vi "standardize CSM Module.vi"(8 "Error In":errorcluster, 11 "CSM-Helper In":refnum<class "CSM-Helper.lvclass">) -> (0 "error out":errorcluster, 3 "CSM-Helper Out":refnum<class "CSM-Helper.lvclass">)   [LabVIEW 2017, in "CSM-Helper.lvclass"]
doc: "### standardize CSM Module.vi\n\n-- <b>Controls</b> --\n- <b>CSM-Helper in</b>: CSMHelper input\n\n-- <b>Indicators</b> --\n- <b>CSM-Helper out</b>: CSMHelper output"
uses:
  CSM-Helper.lvclass
  CSM-Helper.lvclass/CSM-Helper.ctl
  Properties/Read Type.vi
  API/Set Visible Case Frame.vi
  API/Get CaseFrame Reference By CaseName.vi
  API/Stop Undo.vi
  API/Start Undo.vi
  Utility/CSM-Helper Utility.lvlib
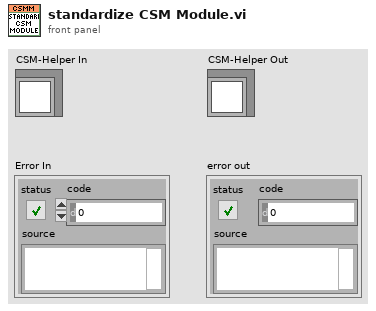
[diagram p1: front panel]
types:
  T1 = enum32{"Invalid", "Standard", "Closed", "Hidden", "Minimized", "Maximized"}
  T2 = enum32{"invalid app kind", "Development System", "Run Time System", "Student Edition", "Embedded LabVIEW", "Evaluation", "Custom"}
  T3 = cluster{"Core":cluster{"Current VI Reference":refnum<vi>, "Close Panel on Exit?":bool}, "Your Boolean data":bool, "Your string data":string}
  T4 = cluster{"Current VI Reference":refnum<vi>, "Close Panel on Exit?":bool}
  T5 = typedef "CSM-Helper Utility.lvlib/CSM Module Type.ctl" = enum16{"Not a CSM", "JKISM", "CSM"}
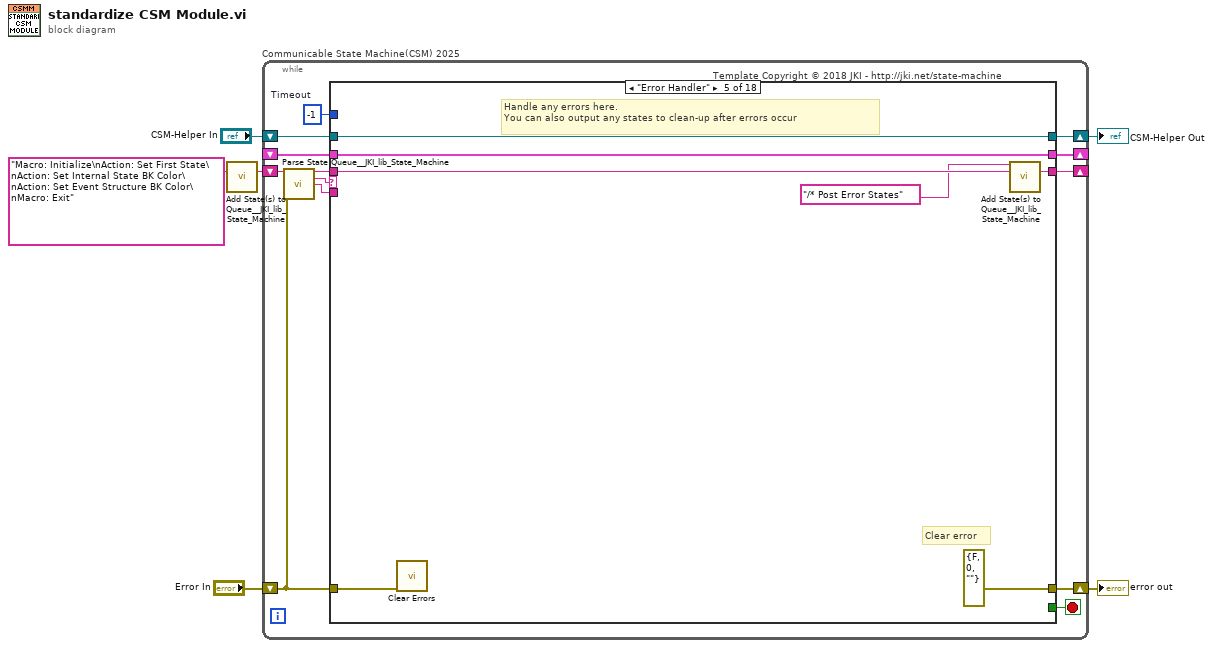
[diagram p0: block diagram]
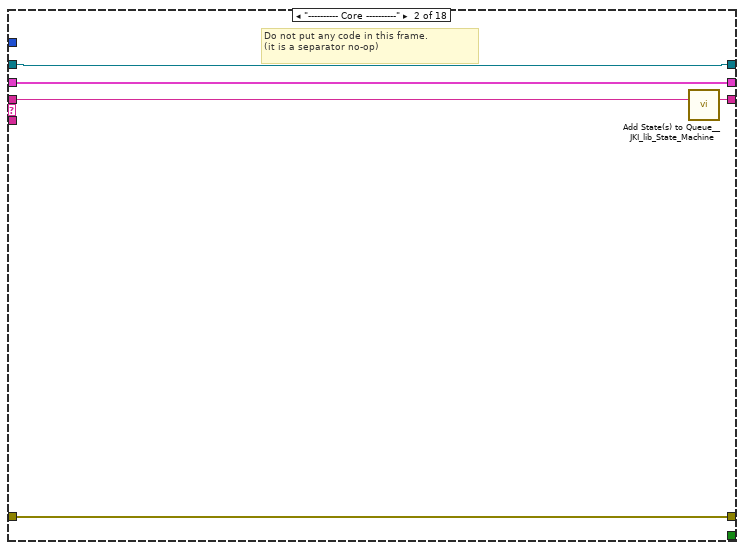
[diagram p3: hidden frame]
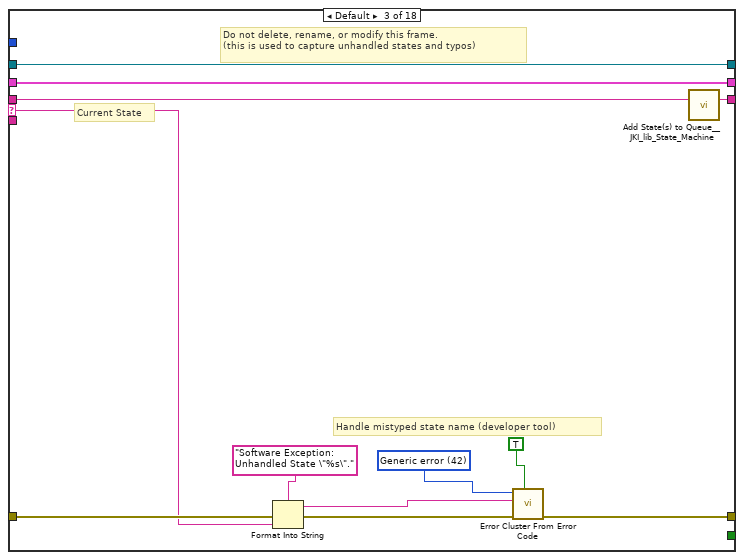
[diagram p4: hidden frame]
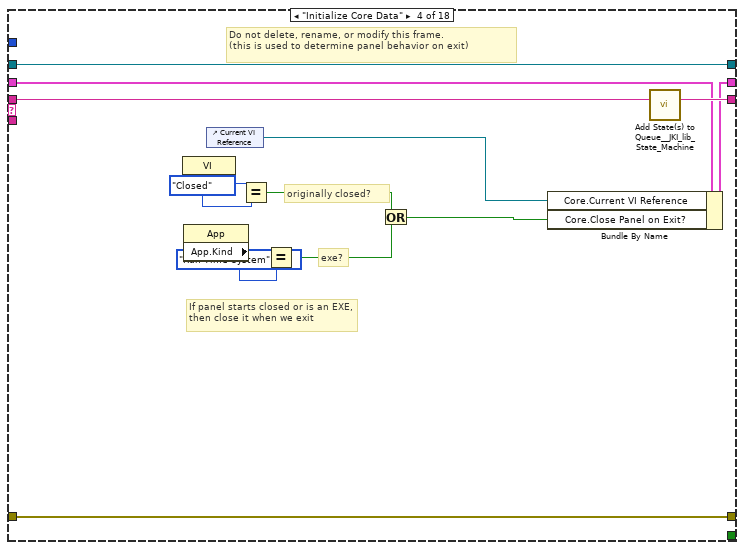
[diagram p5: hidden frame]
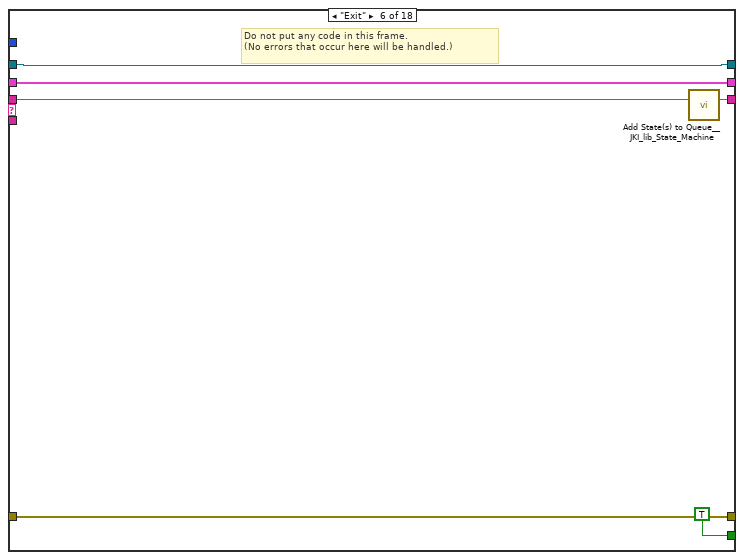
[diagram p6: hidden frame]
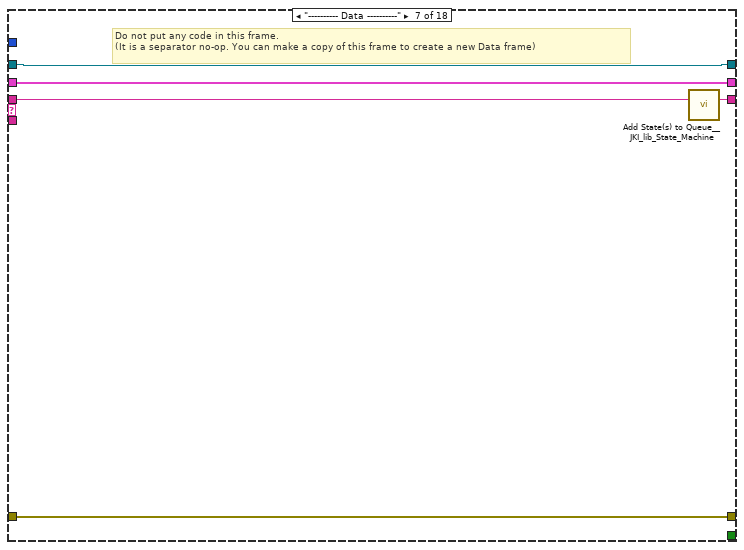
[diagram p7: hidden frame]
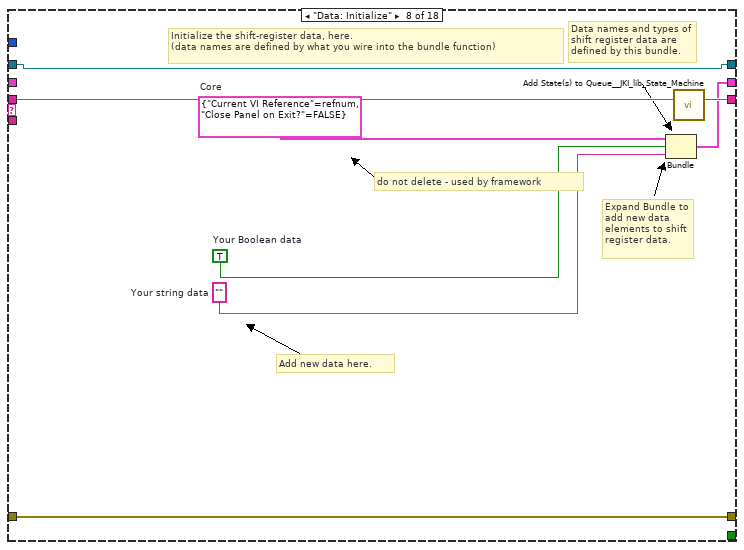
[diagram p8: hidden frame]
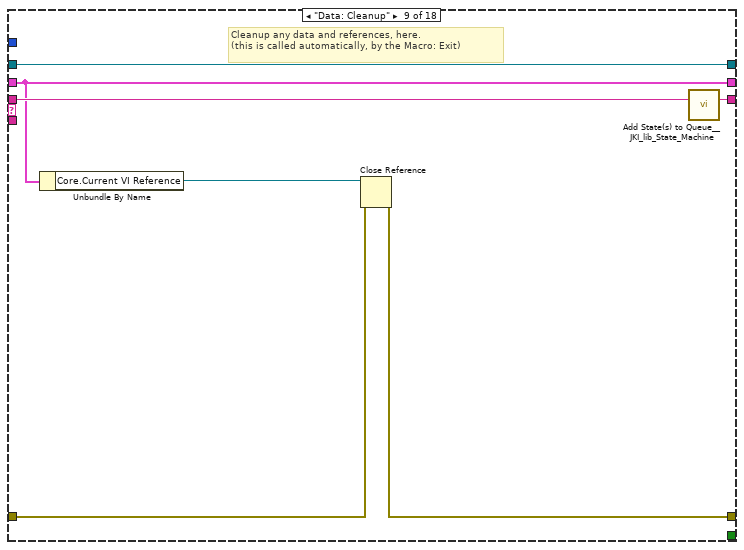
[diagram p9: hidden frame]
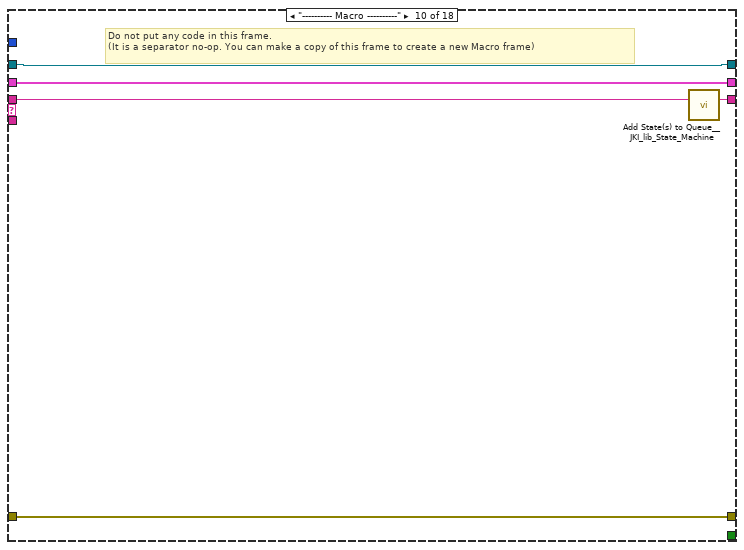
[diagram p10: hidden frame]
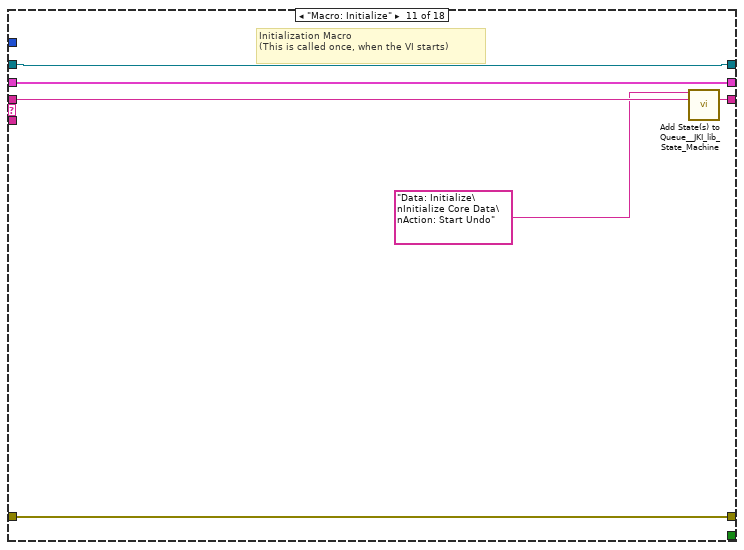
[diagram p11: hidden frame]
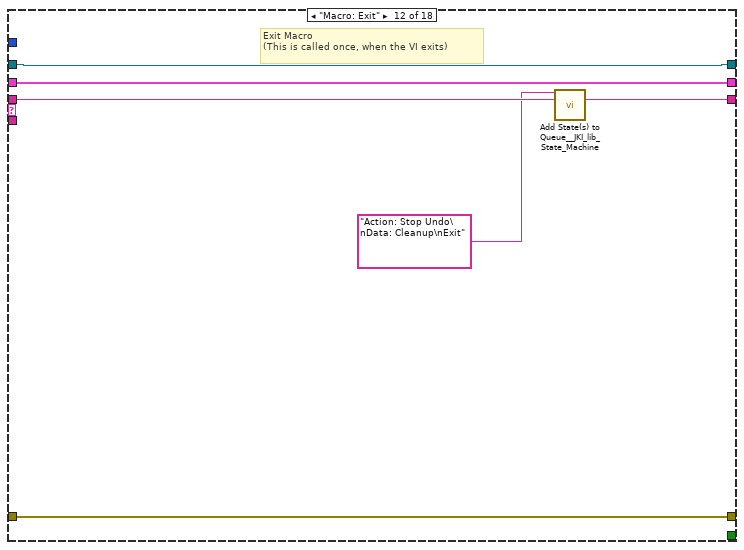
[diagram p12: hidden frame]
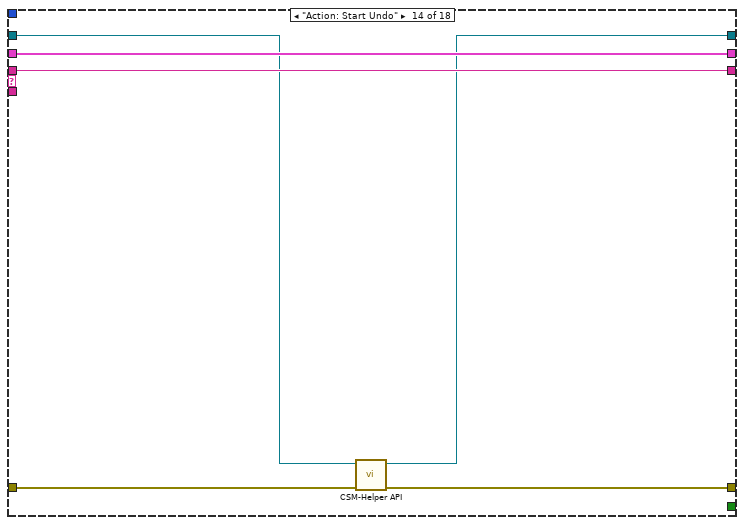
[diagram p14: hidden frame]
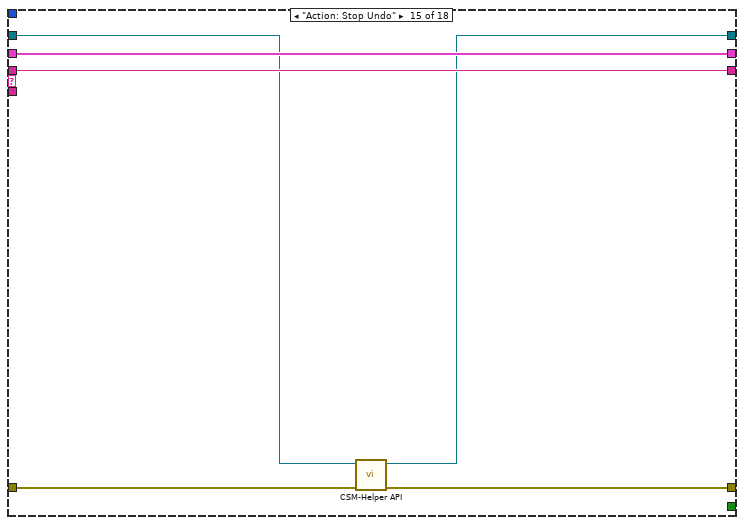
[diagram p15: hidden frame]
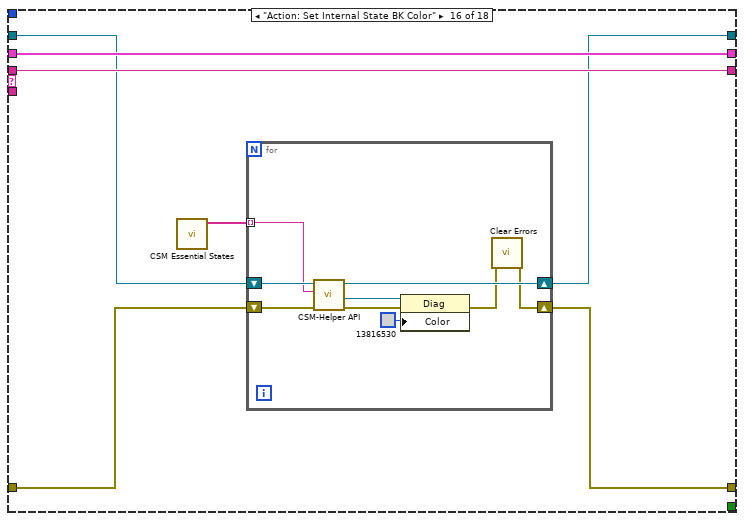
[diagram p16: hidden frame]
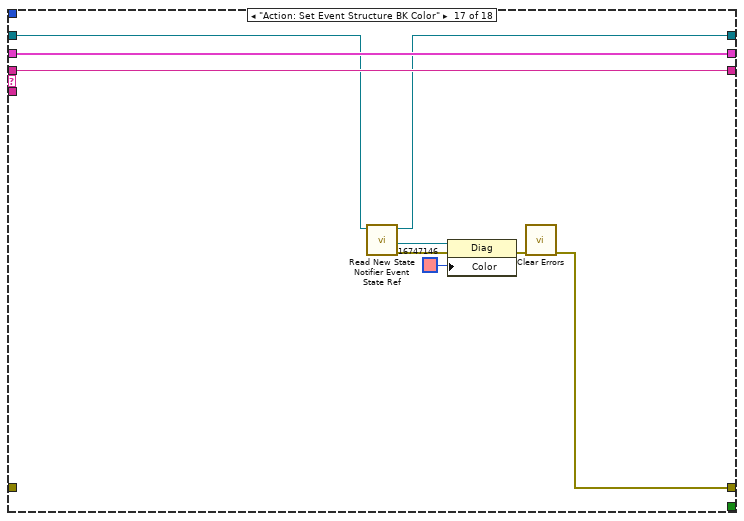
[diagram p17: hidden frame]
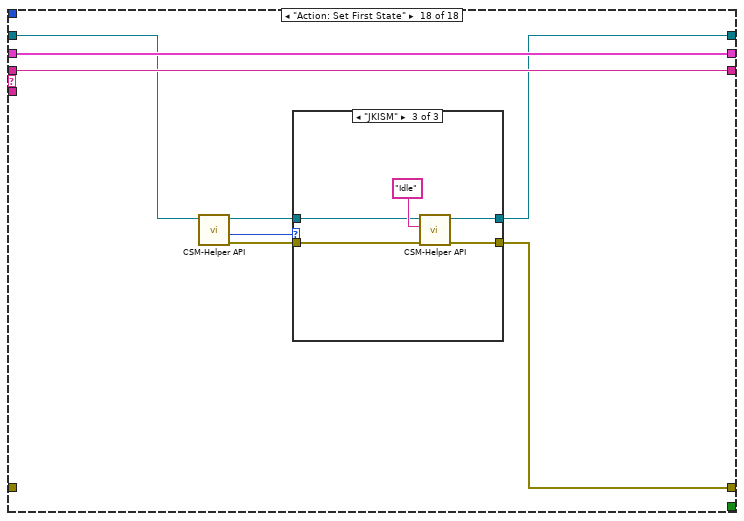
[diagram p18: hidden frame]
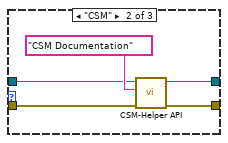
[diagram p20: hidden frame]
diagram:
  n1 = call <vilib>:"Add State(s) to Queue__JKI_lib_State_Machine.vi"("State(s) in (\"\")"="Macro: Initialize\nAction: Set First State\nAction: Set Internal State BK Color\nAction: Set Event Structure BK Color\nMacro: Exit") -> ("States Out"=w6:string)  [unwired: 14 in]
  n2 = while "Communicable State Machine(CSM) 2025" {
    shift-right: [w12] -> _
    shift-left: _ -> [w11]
    shift-right: [w15] -> w3
    shift-left: "Error In" -> [w9]
    shift-right: [w14] -> _
    shift-left: w6 -> [w16]
    shift-right: [w7] -> w1
    shift-left: "CSM-Helper In" -> [w8]
    stop <- w13 stop-if-true
    w10 = -1  # Timeout
    # "Template Copyright © 2018 JKI - http://jki.net/state-machine"
    n3 = call <vilib>:"Parse State Queue__JKI_lib_State_Machine.vi"("State Queue"=w16, "Error In (no error)"=w9) -> ("Remaining States"=w18:string, "Current State"=w19:string, "Arguments"=w17:string)  [unwired: 11 in]
    n4 = case shown="\"Error Handler\"" w19 {
      selector: w19 -> [_ _ w30 _ _ _ _ _ _ _ _ _ _ _ _ _ _ _]
      tunnel: w18 -> [w23 w28 w34 w54 w61 w67 w72 w80 w87 w92 w98 w104 w106 w113 w119 w127 w145 w153]
      tunnel: w17 -> [_ _ _ _ _ _ _ _ _ _ _ _ _ _ _ _ _ _]
      tunnel: w11 -> [w21 w25 w32 w47 w58 w65 w69 _ w82 w89 w95 w101 w107 w114 w120 w126 w144 w152]
      tunnel: [w22 w26 w36 w51 errorcluster {"status"=FALSE, "code"=0, "source"=""} ("error out") w64 w70 w77 w83 w90 w96 w102 w105 w111 w117 w122 w137 w150] -> w15
      tunnel: w9 -> [w22 w26 w35 w51 w57 w64 w70 w77 w84 w90 w96 w102 w105 w112 w118 w123 _ _]
      tunnel: [w23 w27 w33 w53 w60 w66 w71 w79 w86 w91 w97 w103 w106 w113 w119 w127 w145 w153] -> w14
      tunnel: [_ _ _ _ _ TRUE _ _ _ _ _ _ _ _ _ _ _ _] -> w13
      tunnel: [w21 w25 w32 w52 w58 w65 w69 w78 w82 w89 w95 w101 w107 w114 w120 w126 w144 w152] -> w12
      tunnel: w10 -> [_ _ _ _ _ _ _ _ _ _ _ _ _ _ _ _ _ _]
      tunnel: w8 -> [w20 w24 w29 w41 w55 w62 w68 w73 w81 w88 w93 w99 w108 w110 w116 w125 w143 w149]
      tunnel: [w20 w24 w29 w41 w55 w62 w68 w73 w81 w88 w93 w99 w108 w109 w115 w124 w142 w151] -> w7
      frame "", "Event Structure", "Idle" {
        # "executes when the state queue is empty"
      }
      frame "---------- Core ----------" {
        # "Do not put any code in this frame.\n(it is a separator no-op)"
        n5 = call <vilib>:"Add State(s) to Queue__JKI_lib_State_Machine.vi"("State(s) in (\"\")"=w28) -> ("States Out"=w27:string)  [unwired: 14 in]
      }
      frame Default {
        w39 = 42 items=["No error", "Argument error", "Memory is full", "Out of zone", "End of file", "File already open", "Generic file I/O error", "File not found", "File permission error", "Disk is full", "Duplicate path", "Too many files open", "System feature not enabled", "Resource file not found", "Cannot add resource", "Resource not found", "Image not found", "Image memory error", "Pen does not exist", "Config type invalid", "Config token not found", "Config parse error", "Config memory error", "Bad external code format", "Bad external code offset", "External code not present", "Null window", "Destroy window error", "Null menu", "Print aborted", "Bad print record", "Print driver error", "Windows error during printing", "Memory error during printing", "Print dialog error", "Generic print error", "Invalid device refnum", "Device not found", "Device parameter error", "Device unit error", "Cannot open device", "Device call aborted", "Generic error", "Cancelled by user", "Object ID too low", "Object ID too high", "Object not in heap", "Unknown heap", "Unknown object (invalid DefProc)", "Unknown object (DefProc not in table)", "Message out of range", "Invalid (null) method", "Unknown message", "Manager call not supported", "Bad address", "Network operation in progress", "Network operation timed out", "Connection is busy", "Network attribute not supported", "Network error", "Address in use", "System out of memory", "Connection aborted", "Connection refused", "Not connected", "Already connected", "Connection closed", "Initialization error (interapplication manager)", "Bad occurrence", "Wait on unbound occurrence handler", "Occurrence queue overflow", "Datalog type conflict", "Unused", "Unrecognized type (interapplication manager)", "Memory corrupt", "Failed to make temporary DLL", "Old CIN version", "Drag socket not found", "Failed to load drop-object", "Failed to register OLE object", "Failed to release OLE object", "Format specifier type mismatch", "Unknown format specifier", "Too few format specifiers", "Too many format specifiers", "Scan failed", "Newer CIN version", "Error converting to variant", "Runtime menu error", "Password tampered", "Variant attribute not found", "Incompatible variant data type", "Event data is not available", "Event Store is not present", "Occurrence is not found", "Event Queue is not created", "Event info is not available", "Refnum passed is NULL", "Error retrieving Class GUID", "Error retrieving CoClass GUID", "Error retrieving TypeLib GUID.", "Bad built application magic bytes.", "Specific driver is different from the specific driver associated with the Logical Name.", "There is no session opened to the class driver.", "Max Error", "MAX - Error with config objects", "MAX - Error loading configuration", "MAX - Group not supported"]
        # "Current State"
        # "Do not delete, rename, or modify this frame.\n(this is used to capture unhandled states and typos)"
        # "Handle mistyped state name (developer tool)"
        n6 = Format Into String(format string="Software Exception: Unhandled State \"%s\"." ("message"), error in=w35, w30) -> (resulting string=w38:string, error out=w37:errorcluster)  [unwired: 1 in]
        n7 = call <vilib>:"Error Cluster From Error Code.vi"("show call chain? (False)"=TRUE, "error in (no error)"=w37, "error message (\"\")"=w38, "error code (0)"=w39) -> ("error out"=w36:errorcluster)  [unwired: 5 in]
        n8 = call <vilib>:"Add State(s) to Queue__JKI_lib_State_Machine.vi"("State(s) in (\"\")"=w34) -> ("States Out"=w33:string)  [unwired: 14 in]
      }
      frame "Initialize Core Data" {
        # "Do not delete, rename, or modify this frame.\n(this is used to determine panel behavior on exit)"
        # "originally closed?"
        # "exe?"
        # "If panel starts closed or is an EXE, then close it when we exit"
        n9 = property class="VI"() -> ("FP.State"=w44:T1)  [unwired: 2 in, 2 out]
        n10 = property class="App"() -> ("App.Kind"=w50:T2)  [unwired: 2 in, 2 out]
        n11 = control-ref of="Current VI Reference"() -> (w45:refnum<vi>)
        n12 = Equal?(x=w44, y=T1."Closed" ("Front Panel Window:State")) -> (x = y?=w42:bool)
        n13 = Equal?(x=w50, y=T2."Run Time System" ("Application:Kind")) -> (x = y?=w48:bool)
        n14 = Or(x=w42, y=w48) -> (x .or. y?=w46:bool)
        n15 = Bundle By Name(cluster=w47, "Core.Current VI Reference"=w45, "Core.Close Panel on Exit?"=w46) -> (w52:T3)
        n16 = call <vilib>:"Add State(s) to Queue__JKI_lib_State_Machine.vi"("State(s) in (\"\")"=w54) -> ("States Out"=w53:string)  [unwired: 14 in]
      }
      frame "Error Handler" {
        # "Handle any errors here.\nYou can also output any states to clean-up after errors occur"
        # "Clear error"
        n17 = call <vilib>:"Clear Errors.vi"("error in (no error)"=w57) -> ()  [unwired: 5 in, 2 out]
        n18 = call <vilib>:"Add State(s) to Queue__JKI_lib_State_Machine.vi"("State(s) in Front (\"\")"="/* Post Error States", "State(s) in (\"\")"=w61) -> ("States Out"=w60:string)  [unwired: 13 in]
      }
      frame "Exit" {
        # "Do not put any code in this frame.\n(No errors that occur here will be handled.)"
        n19 = call <vilib>:"Add State(s) to Queue__JKI_lib_State_Machine.vi"("State(s) in (\"\")"=w67) -> ("States Out"=w66:string)  [unwired: 14 in]
      }
      frame "---------- Data ----------" {
        # "Do not put any code in this frame.\n(It is a separator no-op. You can make a copy of this frame to create a new Data frame)"
        n20 = call <vilib>:"Add State(s) to Queue__JKI_lib_State_Machine.vi"("State(s) in (\"\")"=w72) -> ("States Out"=w71:string)  [unwired: 14 in]
      }
      frame "Data: Initialize" {
        w74 = T4 {"Current VI Reference"=refnum, "Close Panel on Exit?"=FALSE}  # Core
        w76 = TRUE  # Your Boolean data
        w75 = ""  # Your string data
        # "do not delete - used by framework"
        # "Expand Bundle to add new data elements to shift register data."
        # "Add new data here."
        # "Data names and types of shift register data are defined by this bundle."
        # "Initialize the shift-register data, here.\n(data names are defined by what you wire into the bundle function)"
        n21 = Bundle("Core"=w74, "Your Boolean data"=w76, "Your string data"=w75) -> (w78:T3)  [unwired: 1 in]
        n22 = call <vilib>:"Add State(s) to Queue__JKI_lib_State_Machine.vi"("State(s) in (\"\")"=w80) -> ("States Out"=w79:string)  [unwired: 14 in]
      }
      frame "Data: Cleanup" {
        # "Cleanup any data and references, here.\n(this is called automatically, by the Macro: Exit)"
        n23 = Unbundle By Name(w82) -> ("Core.Current VI Reference"=w85:refnum<vi>)
        n24 = Close Reference(reference=w85, error in (no error)=w84) -> (error out=w83:errorcluster)
        n25 = call <vilib>:"Add State(s) to Queue__JKI_lib_State_Machine.vi"("State(s) in (\"\")"=w87) -> ("States Out"=w86:string)  [unwired: 14 in]
      }
      frame "---------- Macro ----------" {
        # "Do not put any code in this frame.\n(It is a separator no-op. You can make a copy of this frame to create a new Macro frame)"
        n26 = call <vilib>:"Add State(s) to Queue__JKI_lib_State_Machine.vi"("State(s) in (\"\")"=w92) -> ("States Out"=w91:string)  [unwired: 14 in]
      }
      frame "Macro: Initialize" {
        # "Initialization Macro\n(This is called once, when the VI starts)"
        n27 = call <vilib>:"Add State(s) to Queue__JKI_lib_State_Machine.vi"("State(s) in Front (\"\")"="Data: Initialize\nInitialize Core Data\nAction: Start Undo", "State(s) in (\"\")"=w98) -> ("States Out"=w97:string)  [unwired: 13 in]
      }
      frame "Macro: Exit" {
        # "Exit Macro\n(This is called once, when the VI exits)"
        n28 = call <vilib>:"Add State(s) to Queue__JKI_lib_State_Machine.vi"("State(s) in Front (\"\")"="Action: Stop Undo\nData: Cleanup\nExit", "State(s) in (\"\")"=w104) -> ("States Out"=w103:string)  [unwired: 13 in]
      }
      frame "--------- Action -----------" {
      }
      frame "Action: Start Undo" {
        n29 = call-poly "CSM-Helper API.vi"("error in (no error)"=w112, "CSM-Helper in"=w110) -> ("error out"=w111:errorcluster, "CSM-Helper out"=w109:refnum<class "CSM-Helper.lvclass">)  [unwired: 8 in]
      }
      frame "Action: Stop Undo" {
        n30 = call-poly "CSM-Helper API.vi"("error in (no error)"=w118, "CSM-Helper in"=w116) -> ("error out"=w117:errorcluster, "CSM-Helper out"=w115:refnum<class "CSM-Helper.lvclass">)  [unwired: 8 in]
      }
      frame "Action: Set Internal State BK Color" {
        n31 = call "CSM Essential States.vi"() -> ("CSM Essential States"=w121:string[])  [unwired: 11 in]
        n32 = for {
          shift-right: [w135] -> w124
          shift-left: w125 -> [w136]
          shift-right: [w128] -> w122
          shift-left: w123 -> [w133]
          tunnel: w121 -> [w129] mode=indexing
          n33 = call-poly "CSM-Helper API.vi"("error in (no error)"=w133, "CASE"=w129, "CSM-Helper in"=w136) -> ("error out"=w134:errorcluster, "Frame Refs"=w131:refnum<vi>, "CSM-Helper out"=w135:refnum<class "CSM-Helper.lvclass">)  [unwired: 6 in]
          n34 = property class="Diag"(reference=w131, error in=w134, "Color"=u32 13816530) -> (error out=w132:errorcluster)  [unwired: 1 out]
          n35 = call <vilib>:"Clear Errors.vi"("error in (no error)"=w132) -> ("error out"=w128:errorcluster)  [unwired: 5 in, 1 out]
        }
      }
      frame "Action: Set Event Structure BK Color" {
        n36 = call "Read New State Notifier Event State Ref.vi"("CSM-Helper in"=w143) -> ("error out"=w141:errorcluster, "New State Notifier Event State Ref"=w139:refnum<vi>, "CSM-Helper out"=w142:refnum<class "CSM-Helper.lvclass">)  [unwired: 8 in]
        n37 = property class="Diag"(reference=w139, error in=w141, "Color"=u32 16747146) -> (error out=w140:errorcluster)  [unwired: 1 out]
        n38 = call <vilib>:"Clear Errors.vi"("error in (no error)"=w140) -> ("error out"=w137:errorcluster)  [unwired: 5 in, 1 out]
      }
      frame "Action: Set First State" {
        n39 = call-poly "CSM-Helper API.vi"("CSM-Helper in"=w149) -> ("error out"=w147:errorcluster, "Part References.Type"=w146:T5, "CSM-Helper out"=w148:refnum<class "CSM-Helper.lvclass">)  [unwired: 8 in]
        n40 = case shown="\"JKISM\"" w146 {
          tunnel: [w155 w160 w165] -> w151
          tunnel: [w154 w159 w164] -> w150
          tunnel: w148 -> [w155 w157 w162]
          tunnel: w147 -> [w154 w156 w161]
          frame "Not a CSM", Default {
          }
          frame "CSM" {
            n41 = call-poly "CSM-Helper API.vi"("error in (no error)"=w156, "element"="CSM Documentation", "CSM-Helper in"=w157) -> ("error out"=w159:errorcluster, "CSM-Helper out"=w160:refnum<class "CSM-Helper.lvclass">)  [unwired: 7 in]
          }
          frame "JKISM" {
            n42 = call-poly "CSM-Helper API.vi"("error in (no error)"=w161, "element"="Idle", "CSM-Helper in"=w162) -> ("error out"=w164:errorcluster, "CSM-Helper out"=w165:refnum<class "CSM-Helper.lvclass">)  [unwired: 7 in]
          }
        }
      }
    }
  }
  "error out" <- w3
  "CSM-Helper Out" <- w1
